vi "Logic.vi"(6 "DestinationReached":bool, 8 "D":bool, 9 "C":bool, 10 "B":bool, 11 "A":bool) -> (2 "State":string)   [LabVIEW 2017]
panel:
  out "D":bool
  out "C":bool
  out "B":bool
  out "A":bool
  out "~D":bool
  out "~C":bool
  out "~B":bool
  out "~A":bool
  # "This vi takes in the logic lines produced by testing greater comparisons on target current and past location data.\nThat logic is then put through a boolean POS circuit which results in a decision string that tells the robot what its\nnext action should be to get it closer to the target."
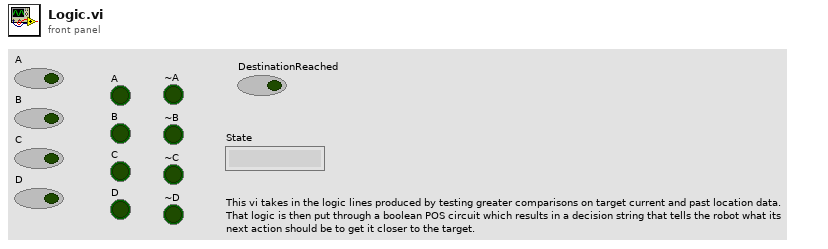
[diagram p1: front panel]
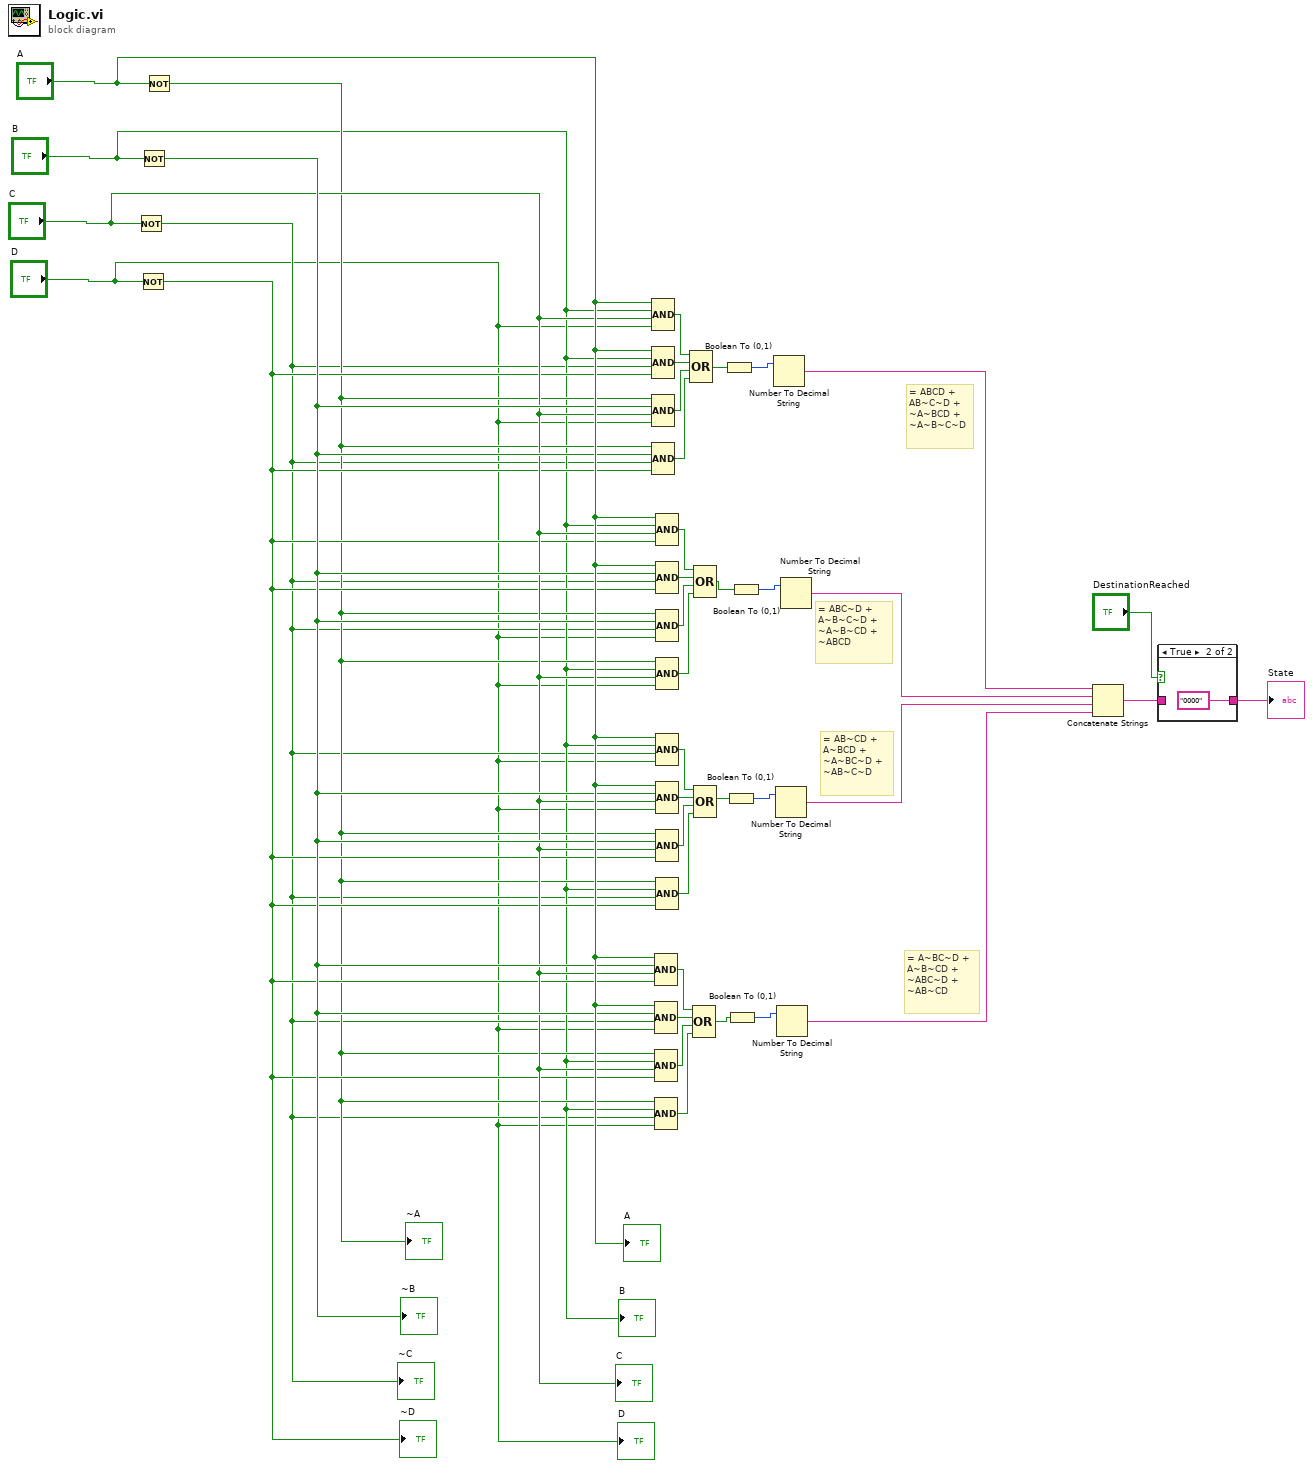
[diagram p0: block diagram]
diagram:
  # "= A~BC~D + A~B~CD + ~ABC~D + ~AB~CD"
  # "= AB~CD + A~BCD + ~A~BC~D + ~AB~C~D"
  # "= ABC~D + A~B~C~D + ~A~B~CD + ~ABCD"
  # "= ABCD + AB~C~D + ~A~BCD + ~A~B~C~D"
  n1 = Not(x="C") -> (.not. x?=w17:bool)
  "~C" <- w17
  n2 = Not(x="D") -> (.not. x?=w20:bool)
  "~D" <- w20
  n3 = Not(x="B") -> (.not. x?=w22:bool)
  "~B" <- w22
  n4 = Not(x="A") -> (.not. x?=w19:bool)
  "~A" <- w19
  n5 = Compound Arithmetic op=AND("A", "B", "C", "D") -> (w39:bool)
  n6 = Compound Arithmetic op=AND("A", "B", w17, w20) -> (w36:bool)
  n7 = Compound Arithmetic op=AND(w19, w22, "C", "D") -> (w37:bool)
  n8 = Compound Arithmetic op=AND(w19, w22, w17, w20) -> (w38:bool)
  n9 = Compound Arithmetic op=AND("A", w22, "C", w20) -> (w27:bool)
  n10 = Compound Arithmetic op=AND("A", w22, w17, "D") -> (w25:bool)
  n11 = Compound Arithmetic op=AND(w19, "B", "C", w20) -> (w24:bool)
  n12 = Compound Arithmetic op=AND(w19, "B", w17, "D") -> (w26:bool)
  n13 = Compound Arithmetic op=AND("A", "B", "C", w20) -> (w35:bool)
  n14 = Compound Arithmetic op=AND("A", w22, w17, w20) -> (w33:bool)
  n15 = Compound Arithmetic op=AND(w19, w22, w17, "D") -> (w32:bool)
  n16 = Compound Arithmetic op=AND(w19, "B", "C", "D") -> (w34:bool)
  n17 = Compound Arithmetic op=AND("A", "B", w17, "D") -> (w31:bool)
  n18 = Compound Arithmetic op=AND("A", w22, "C", "D") -> (w29:bool)
  n19 = Compound Arithmetic op=AND(w19, w22, "C", w20) -> (w28:bool)
  n20 = Compound Arithmetic op=AND(w19, "B", w17, w20) -> (w30:bool)
  n21 = Compound Arithmetic op=OR(w39, w36, w37, w38) -> (w15:bool)
  n22 = Compound Arithmetic op=OR(w27, w25, w24, w26) -> (w6:bool)
  n23 = Compound Arithmetic op=OR(w35, w33, w32, w34) -> (w11:bool)
  n24 = Compound Arithmetic op=OR(w31, w29, w28, w30) -> (w8:bool)
  n25 = Boolean To (0,1)(Boolean=w15) -> (0, 1=w14:i16)
  n26 = Boolean To (0,1)(Boolean=w8) -> (0, 1=w9:i16)
  n27 = Boolean To (0,1)(Boolean=w6) -> (0, 1=w7:i16)
  n28 = Boolean To (0,1)(Boolean=w11) -> (0, 1=w12:i16)
  n29 = Number To Decimal String(number=w14) -> (decimal integer string=w13:string)  [unwired: 1 in]
  n30 = Number To Decimal String(number=w9) -> (decimal integer string=w5:string)  [unwired: 1 in]
  n31 = Number To Decimal String(number=w7) -> (decimal integer string=w4:string)  [unwired: 1 in]
  n32 = Number To Decimal String(number=w12) -> (decimal integer string=w10:string)  [unwired: 1 in]
  n33 = Concatenate Strings(w13, w10, w5, w4) -> (w2:string)
  n34 = case shown="True" "DestinationReached" {
    tunnel: [w40 "0000"] -> w3
    tunnel: w2 -> [w40 _]
    frame False {
    }
    frame True {
    }
  }
  "State" <- w3
  "A" <- "A"
  "B" <- "B"
  "C" <- "C"
  "D" <- "D"
